vi "UpdateList.vi"(6 "DetectArray":cluster{"T0":u8, "T1":u8, "br_selfdef":T1}[](array[cluster]) {"br_selfdef"."PHSEG2" items=["CAN_BIT_1TQ"=1, "CAN_BIT_2TQ"=2, "CAN_BIT_3TQ"=3, "CAN_BIT_4TQ"=4, "CAN_BIT_5TQ"=5, "CAN_BIT_6TQ"=6, "CAN_BIT_7TQ"=7, "CAN_BIT_8TQ"=8]; "br_selfdef"."PHSEG1" items=["CAN_BIT_1TQ"=1, "CAN_BIT_2TQ"=2, "CAN_BIT_3TQ"=3, "CAN_BIT_4TQ"=4, "CAN_BIT_5TQ"=5, "CAN_BIT_6TQ"=6, "CAN_BIT_7TQ"=7, "CAN_BIT_8TQ"=8]; "br_selfdef"."PRSEG" items=["CAN_BIT_1TQ"=1, "CAN_BIT_2TQ"=2, "CAN_BIT_3TQ"=3, "CAN_BIT_4TQ"=4, "CAN_BIT_5TQ"=5, "CAN_BIT_6TQ"=6, "CAN_BIT_7TQ"=7, "CAN_BIT_8TQ"=8]; "br_selfdef"."PHS2_SEL" items=["由相位缓冲段1时间指定", "可编程"]; "br_selfdef"."SAM" items=["采样一次", "采样三次"]; "br_selfdef"."BRP" items=["1"=1, "2"=2, "3"=3, "4"=4, "5"=5, "6"=6, "7"=7, "8"=8, "9"=9, "10"=10, "11"=11, "12"=12, "13"=13, "14"=14, "15"=15, "16"=16, "17"=17, "18"=18, "19"=19, "20"=20, "21"=21, "22"=22, "23"=23, "24"=24, "25"=25, "26"=26, "27"=27, "28"=28, "29"=29, "30"=30, "31"=31, "32"=32, "33"=33, "34"=34, "35"=35, "36"=36, "37"=37, "38"=38, "39"=39, "40"=40, "41"=41, "42"=42, "43"=43, "44"=44, "45"=45, "46"=46, "47"=47, "48"=48, "49"=49, "50"=50, "51"=51, "52"=52, "53"=53, "54"=54, "55"=55, "56"=56, "57"=57, "58"=58, "59"=59, "60"=60, "61"=61, "62"=62, "63"=63, "64"=64]; "br_selfdef"."SJW" items=["1TQ"=1, "2TQ"=2, "3TQ"=3, "4TQ"=4]; "br_selfdef"."SYN(nouse)" items=["CAN_BIT_1TQ"=1]}, 7 "Operation":u8, 9 "VI引用句柄":refnum<vi>, 10 "Baud Rate":u32, 11 "list":refnum<vi>) -> (3 "list out":refnum<vi>)   [LabVIEW 2011]
uses:
  VIs/Baud rate Self Define.ctl
panel:
  # "OP=0正在进行\n=1，匹配\n=2，错误\n=3，Clear并开始"
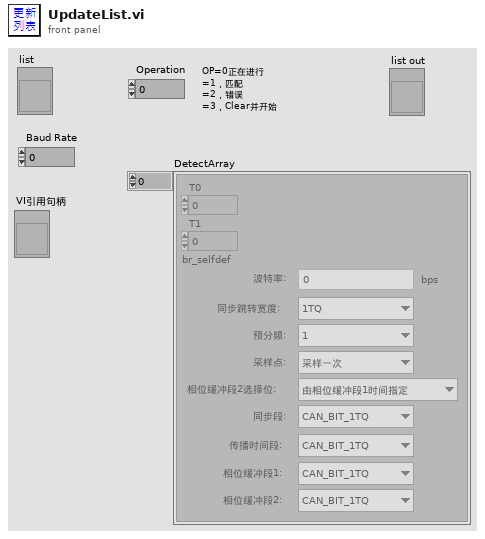
[diagram p1: front panel]
types:
  T1 = typedef "Baud rate Self Define.ctl" = cluster{"BAUD":u32, "SJW":u8, "BRP":u8, "SAM":u8, "PHS2_SEL":u8, "SYN(nouse)":u8, "PRSEG":u8, "PHSEG1":u8, "PHSEG2":u8}
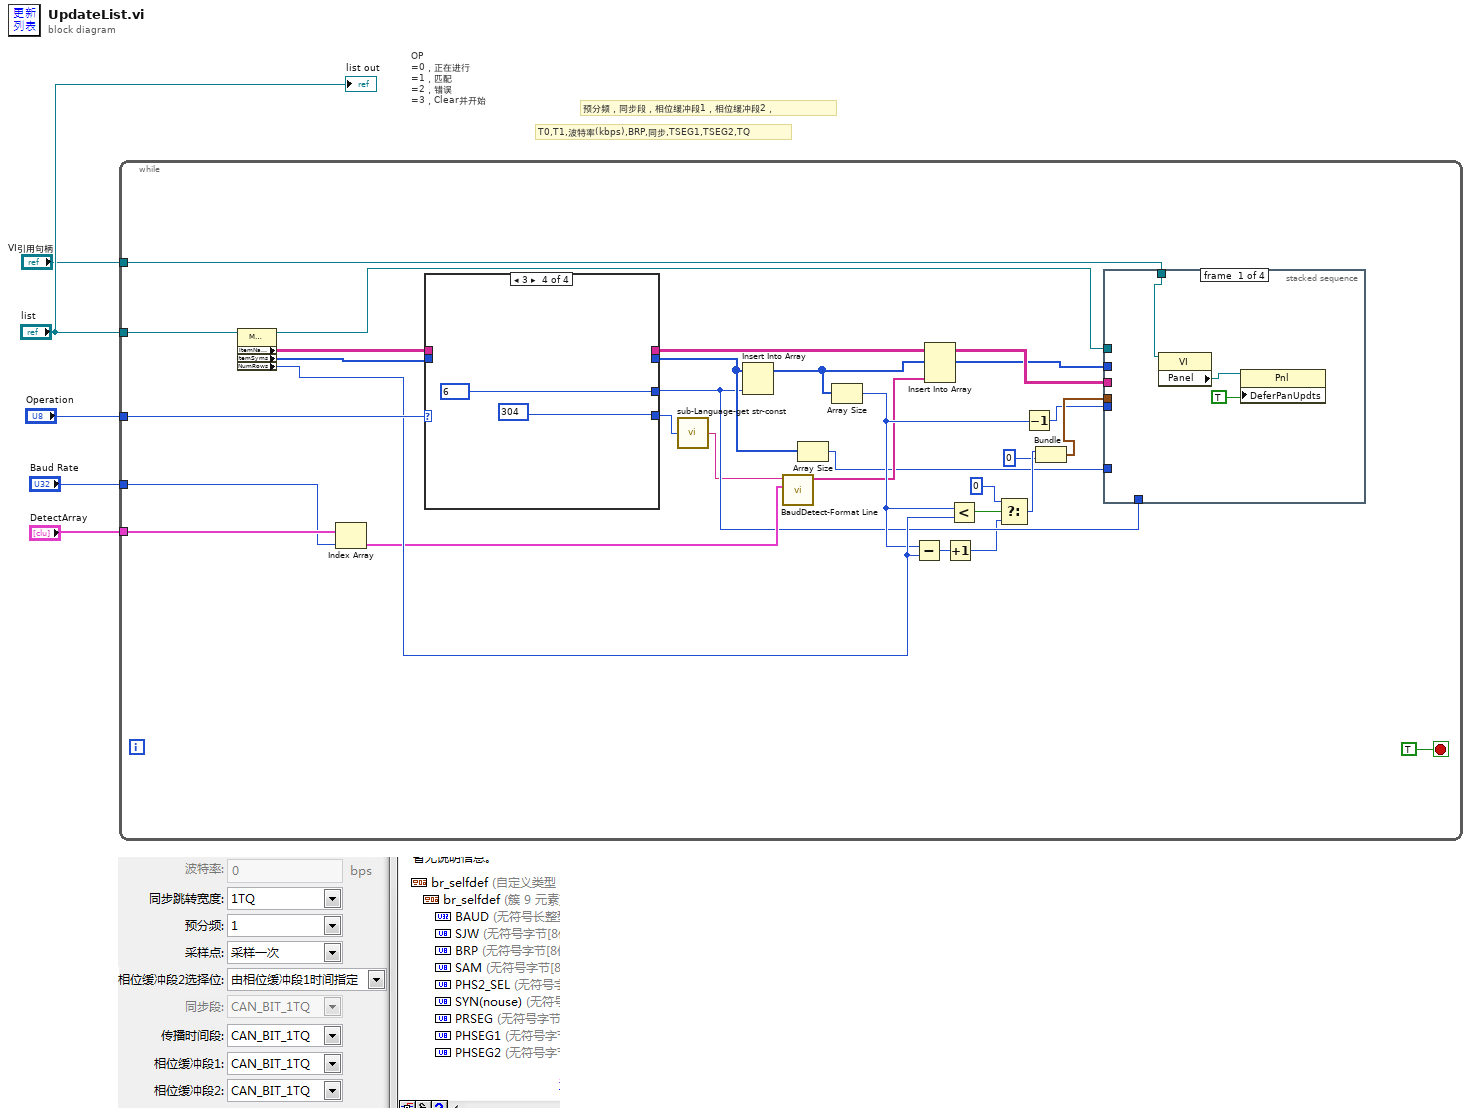
[diagram p0: block diagram]
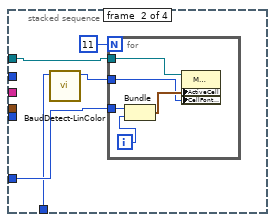
[diagram p2: hidden frame]
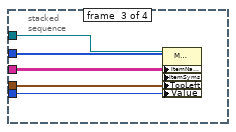
[diagram p3: hidden frame]
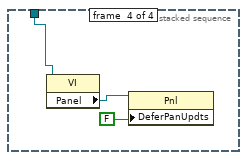
[diagram p4: hidden frame]
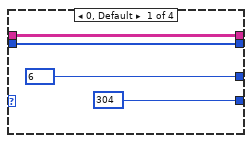
[diagram p5: hidden frame]
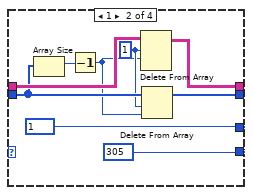
[diagram p6: hidden frame]
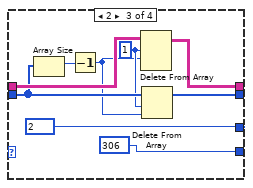
[diagram p7: hidden frame]
diagram:
  # "预分频，同步段，相位缓冲段1，相位缓冲段2，"
  # "T0,T1,波特率(kbps),BRP,同步,TSEG1,TSEG2,TQ"
  # "OP\n=0，正在进行\n=1，匹配\n=2，错误\n=3，Clear并开始"
  n1 = while {
    tunnel: "list" -> [w34]
    tunnel: "DetectArray" -> [w33]
    tunnel: "Baud Rate" -> [w32]
    tunnel: "Operation" -> [w30]
    tunnel: "VI引用句柄" -> [w26]
    stop <- TRUE stop-if-true
    n2 = property class="MCListbox (严格)"(reference=w34) -> (reference out=w14:refnum<vi>, "ItemNames"=w16:string[][], "ItemSyms"=w15:i32[], "NumRows"=w27:u32)  [unwired: 1 in, 1 out]
    n3 = Index Array(array=w33, index=w32) -> (element=w12:cluster{"T0":u8, "T1":u8, "br_selfdef":T1})
    n4 = case shown="3" w30 {
      tunnel: w16 -> [w59 w67 w76 _]
      tunnel: [w59 w65 w74 _] -> w25
      tunnel: w15 -> [w58 w64 w73 _]
      tunnel: [w58 w61 w70 _] -> w11
      tunnel: [6 1 2 6] -> w9
      tunnel: [u32 304 ("sid") u32 305 ("sid") u32 306 ("sid") u32 304 ("sid")] -> w7
      frame 0, Default {
      }
      frame 1 {
        w63 = 1 ("长度")
        n5 = Array Size(array=w64) -> (size(s)=w66:i32)
        n6 = Decrement(x=w66) -> (x-1=w62:i32)
        n7 = Delete From Array(array=w67, length=w63, index (row)=w62) -> (array with subset deleted=w65:string[][])  [unwired: 1 in, 1 out]
        n8 = Delete From Array(array=w64, length=w63, index=w62) -> (array with subset deleted=w61:i32[])  [unwired: 1 out]
      }
      frame 2 {
        w72 = 1 ("长度")
        n9 = Array Size(array=w73) -> (size(s)=w75:i32)
        n10 = Decrement(x=w75) -> (x-1=w71:i32)
        n11 = Delete From Array(array=w76, length=w72, index (row)=w71) -> (array with subset deleted=w74:string[][])  [unwired: 1 in, 1 out]
        n12 = Delete From Array(array=w73, length=w72, index=w71) -> (array with subset deleted=w70:i32[])  [unwired: 1 out]
      }
      frame 3 {
      }
    }
    n13 = call "sub-Language-get str-const.vi"("sid"=w7) -> ("str"=w6:string)
    n14 = Insert Into Array(array=w11, new element=w9) -> (w28:i32[])  [unwired: 1 in]
    n15 = call "BaudDetect-Format Line.vi"("Information"=w12, "Status"=w6) -> ("Line Array"=w13:string[])  [unwired: 9 in]
    n16 = Array Size(array=w11) -> (size(s)=w10:i32)
    n17 = Array Size(array=w28) -> (size(s)=w20:i32)
    n18 = Subtract(x=w20, y=w27) -> (x-y=w22:u32)
    n19 = Insert Into Array(array=w25, new element=w13) -> (w29:string[][])  [unwired: 2 in]
    n20 = Increment(x=w22) -> (x+1=w8:u32)
    n21 = Less?(x=w20, y=w27) -> (x < y?=w24:bool)
    n22 = Select(t=u32 0 ("Column"), s=w24, f=w8) -> (s? t:f=w19:u32)
    n23 = Decrement(x=w20) -> (x-1=w17:i32)
    n24 = Bundle("Column"=w19, "Row"=u32 0) -> (w21:cluster{"Column":u32, "Row":u32})  [unwired: 1 in]
    n25 = stacked-sequence {
      tunnel: w21 -> [_ _ w52 _]
      tunnel: w29 -> [_ _ w51 _]
      tunnel: w28 -> [_ _ w50 _]
      tunnel: w17 -> [_ _ w49 _]
      tunnel: w14 -> [_ w42 w48 _]
      tunnel: w26 -> [w37 _ _ w53]
      tunnel: w10 -> [_ w40 _ _]
      tunnel: w9 -> [_ w39 _ _]
      frame #0 {
        n26 = property class="VI"(reference=w37) -> ("Panel"=w36:refnum<vi>)  [unwired: 1 in, 2 out]
        n27 = property class="Pnl"(reference=w36, "DeferPanUpdts"=TRUE ("延迟前面板更新")) -> ()  [unwired: 1 in, 2 out]
      }
      frame #1 {
        n28 = call "BaudDetect-LinColor.vi"("项符号"=w39) -> ("行颜色"=w38:u32)  [unwired: 10 in]
        n29 = for {
          N: 11 -> [_]
          tunnel: w42 -> [w47]
          tunnel: w40 -> [w46]
          tunnel: w38 -> [w43]
          i -> [w45]
          n30 = Bundle(w46, w45) -> (w44:cluster{i32, i32})  [unwired: 1 in]
          n31 = property class="MCListbox (严格)"(reference=w47, "ActiveCell"=w44, "CellFontColor"=w43) -> ()  [unwired: 1 in, 2 out]
        }
      }
      frame #2 {
        n32 = property class="MCListbox (严格)"(reference=w48, "ItemNames"=w51, "ItemSyms"=w50, "TopLeft"=w52, "Value"=w49) -> ()  [unwired: 1 in, 2 out]
      }
      frame #3 {
        n33 = property class="VI"(reference=w53) -> ("Panel"=w55:refnum<vi>)  [unwired: 1 in, 2 out]
        n34 = property class="Pnl"(reference=w55, "DeferPanUpdts"=FALSE ("延迟前面板更新")) -> ()  [unwired: 1 in, 2 out]
      }
    }
  }
  "list out" <- "list"
